vi "Build Context Menu.vi"(8 "error in (no error)":errorcluster, 10 "MenuRef":refnum<k9>, 11 "HIJ IMAQdx Display in":refnum<class "HIJ IMAQdx Display.lvclass">) -> (0 "error out":errorcluster, 2 "MenuRef out":refnum<k9>, 3 "HIJ IMAQdx Display out":refnum<class "HIJ IMAQdx Display.lvclass">)   [LabVIEW 2020, in "HIJ IMAQdx Display.lvlib" / "HIJ IMAQdx Display.lvclass"]
uses:
  HIJ IMAQdx Display.lvclass
  HIJ IMAQdx Display.lvclass/HIJ IMAQdx Display.ctl
  HIJ Vision Display/HIJ Vision Display/HIJ Vision Display.lvclass
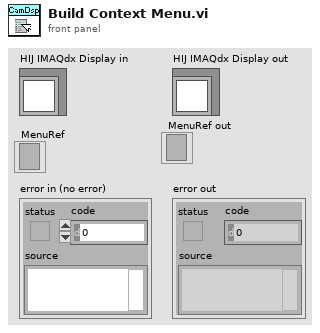
[diagram p1: front panel]
types:
  T1 = typedef "IMAQ Image.ctl" = refnum<image>
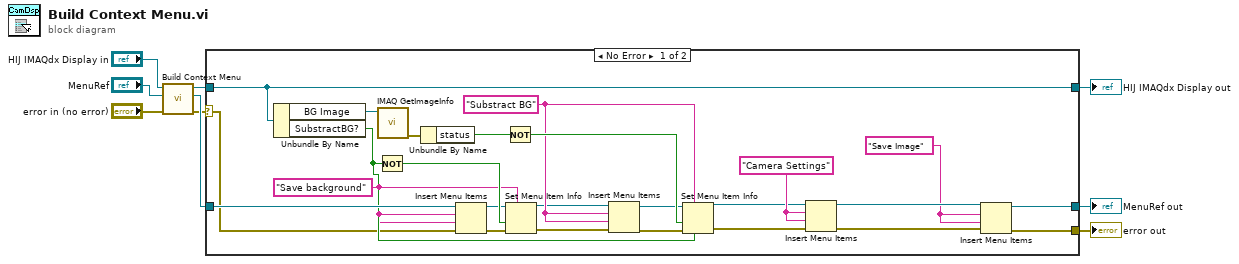
[diagram p0: block diagram]
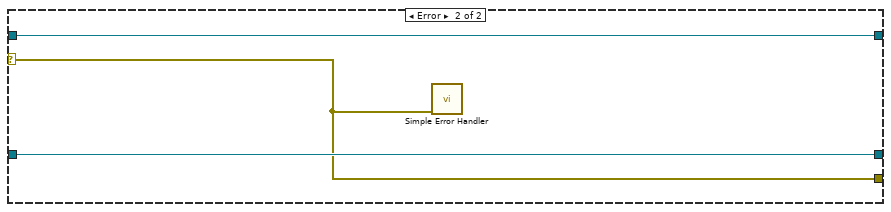
[diagram p2: hidden frame]
diagram:
  n1 = call-parent "Build Context Menu.vi"("error in (no error)"="error in (no error)", "MenuRef"="MenuRef", "HIJ Vision Display in"="HIJ IMAQdx Display in") -> ("error out"=w2:errorcluster, "MenuRef out"=w5:refnum<k9>, "HIJ Vision Display out"=w6:refnum<class "HIJ IMAQdx Display.lvclass">)  [unwired: 6 in]
  n2 = case shown="No Error" w2 {
    selector: w2 -> [w24 w35]
    tunnel: w6 -> [w28 w36]
    tunnel: w5 -> [w29 w37]
    tunnel: [w11 w37] -> w4
    tunnel: [w10 w35] -> w3
    tunnel: [w28 w36] -> w1
    frame No Error {
      w12 = "Save Image" ("item tag")
      w17 = "Camera Settings" ("item tag")
      w22 = "Substract BG" ("item tag")
      w25 = "Save background" ("item tag")
      n3 = Unbundle By Name(w28) -> ("BG Image"=w30:T1, "SubstractBG?"=w27:bool)
      n4 = Not(x=w27) -> (.not. x?=w31:bool)
      n5 = call "IMAQ GetImageInfo"("Image"=w30) -> ("error out"=w33:errorcluster)  [unwired: 3 in, 7 out]
      n6 = Unbundle By Name(w33) -> ("status"=w32:bool)
      n7 = Insert Menu Items(6:w24, 7:w25, 8:w25, 9:w29) -> (0:w23:errorcluster, 3:w26:refnum<k9>)  [unwired: 2 in, 1 out]
      n8 = Not(x=w32) -> (.not. x?=w34:bool)
      n9 = Set Menu Item Info(7:w25, 8:w23, 9:w31, 11:w26) -> (0:w20:errorcluster, 3:w21:refnum<k9>)  [unwired: 3 in]
      n10 = Insert Menu Items(6:w20, 7:w22, 8:w22, 9:w21) -> (0:w18:errorcluster, 3:w19:refnum<k9>)  [unwired: 2 in, 1 out]
      n11 = Set Menu Item Info(6:w27, 7:w22, 8:w18, 9:w34, 11:w19) -> (0:w15:errorcluster, 3:w16:refnum<k9>)  [unwired: 2 in]
      n12 = Insert Menu Items(6:w15, 7:w17, 8:w17, 9:w16) -> (0:w13:errorcluster, 3:w14:refnum<k9>)  [unwired: 2 in, 1 out]
      n13 = Insert Menu Items(6:w13, 7:w12, 8:w12, 9:w14) -> (0:w10:errorcluster, 3:w11:refnum<k9>)  [unwired: 2 in, 1 out]
    }
    frame Error {
      n14 = call <vilib>:"Simple Error Handler.vi"("error in (no error)"=w35) -> ()  [unwired: 4 in, 5 out]
    }
  }
  "error out" <- w3
  "HIJ IMAQdx Display out" <- w1
  "MenuRef out" <- w4
